vi "test_serialize_deserialize.vi"   [LabVIEW 2020, in "Ethernet Frame.lvlib"]
doc: "Version 0.1"
uses:
  <vilib>/ADAS Record/CustomDataTypes/Ethernet Frame/Ethernet Frame.lvlib
  <vilib>/addons/_JKI Toolkits/Caraya/classes/Test/Test.lvclass
  <vilib>/addons/_JKI Toolkits/Caraya/classes/Assert/Assert.lvclass
  <vilib>/ADAS Record/CustomDataTypes/Ethernet Frame/Process Data.ctl
  <vilib>/ADAS Record/CustomDataTypes/Ethernet Frame/Serialize Data.vi
  <vilib>/ADAS Record/CustomDataTypes/Ethernet Frame/Deserialize Data.vi
types:
  T1 = typedef "Ethernet Frame.lvlib/Process Data.ctl" = cluster{"Time Stamp":timestamp, "Source":u64, "Destination":u64, "EtherType":u16, "Payload":u8[]}
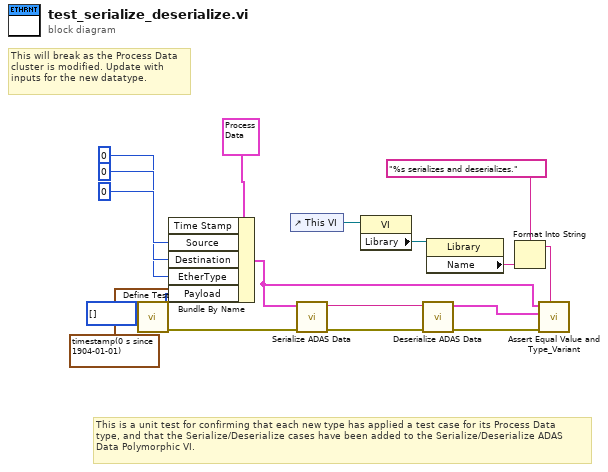
[diagram p0: block diagram]
diagram:
  # "This will break as the Process Data\ncluster is modified. Update with\ninputs for the new datatype."
  # "This is a unit test for confirming that each new type has applied a test case for its Process Data\ntype, and that the Serialize/Deserialize cases have been added to the Serialize/Deserialize ADAS\nData Polymorphic VI."
  n1 = call <vilib>:"Define Test.vi"() -> ("error out"=w12:errorcluster)  [unwired: 11 in]
  n2 = Bundle By Name "Bundle By Name"(cluster=T1 {"Time Stamp"=timestamp(0 s since 1904-01-01), "Source"=0, "Destination"=0, "EtherType"=0, "Payload"=[]} ("Process Data in"), "Time Stamp"=timestamp(0 s since 1904-01-01), "Source"=u64 0, "Destination"=u64 0, "EtherType"=u16 0, "Payload"=u8[] []) -> (w6:T1)
  n3 = control-ref of="This VI"() -> (w17:refnum<vi>)
  n4 = call-poly <vilib>:"Serialize ADAS Data.vi"("error in (no error)"=w12, "Process Data"=w6) -> ("error out"=w11:errorcluster, "Flat Data out"=w10:string)  [unwired: 8 in]
  n5 = property class="VI"(reference=w17) -> ("Library"=w16:refnum<vi>)  [unwired: 1 in, 2 out]
  n6 = call-poly <vilib>:"Deserialize ADAS Data.vi"("error in (no error)"=w11, "Flat Data in"=w10) -> ("error out"=w8:errorcluster, "Process Data out"=w9:T1)  [unwired: 8 in]
  n7 = property class="Library"(reference=w16) -> ("Name"=w14:string)  [unwired: 1 in, 2 out]
  n8 = Format Into String(format string="%s serializes and deserializes.", w14) -> (resulting string=w13:string)  [unwired: 2 in, 1 out]
  n9 = call <vilib>:"Assert Equal Value and Type_Variant.vi"("Label"=w13, "error in (no error)"=w8, "Y"=w9, "X"=w6) -> ()  [unwired: 7 in, 1 out]
